vi "lab2(whithsubvi;works).vi"() -> ()   [LabVIEW 2016]
panel:
  out "2D Picture":picture
  in  "SwapGB":bool
  in  "SwapRB":bool
  in  "SwapRG":bool
  in  "Original":bool
  in  "ImagePath":path
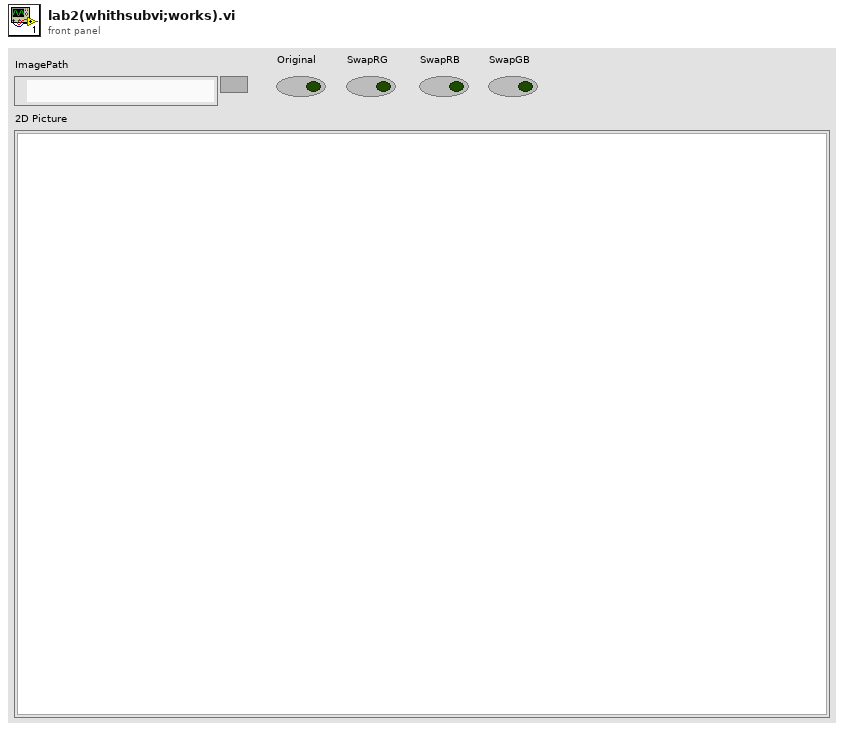
[diagram p1: front panel]
types:
  T1 = typedef "imagedata.ctl" = cluster{"image type":i32, "image depth":i32, "image":u8[], "mask":u8[], "colors":u32[], "Rectangle":cluster{"left":i16, "top":i16, "right":i16, "bottom":i16}}
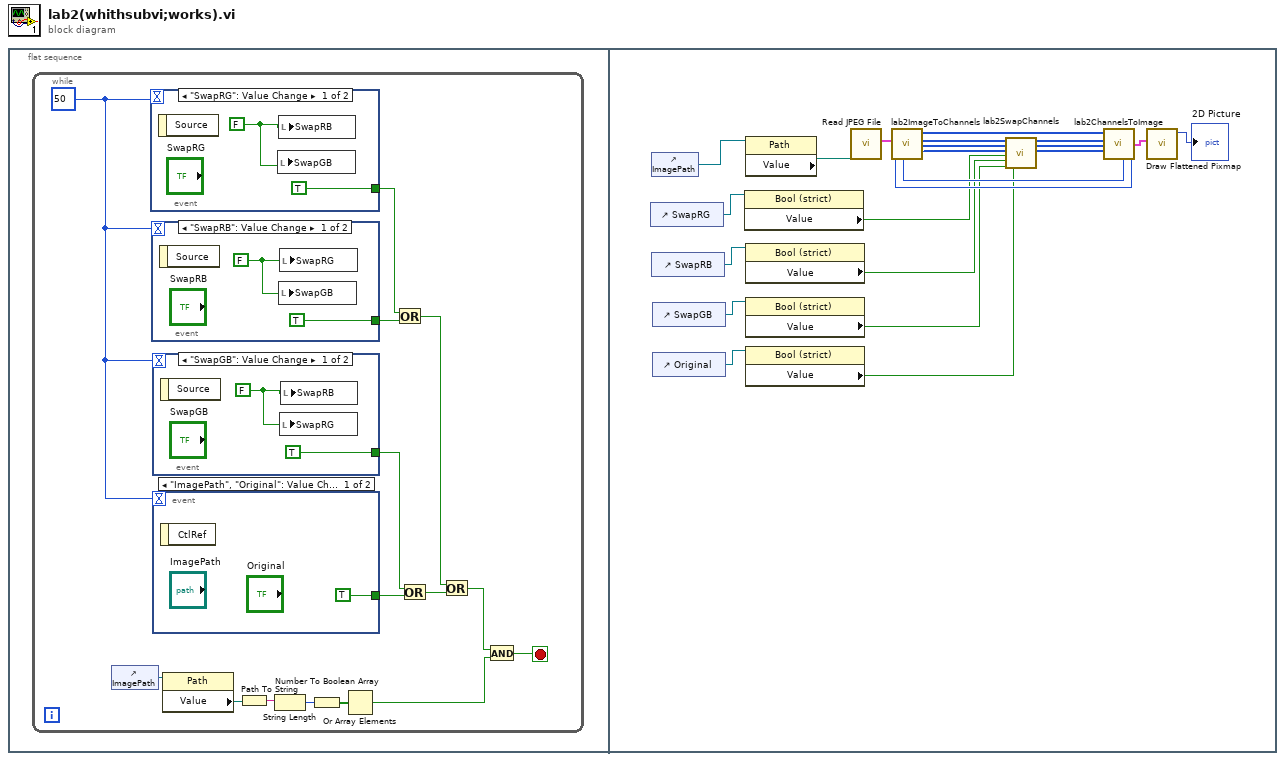
[diagram p0: block diagram]
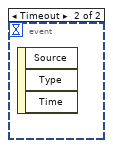
[diagram p2: hidden frame]
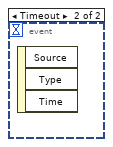
[diagram p3: hidden frame]
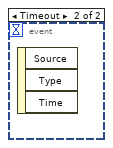
[diagram p4: hidden frame]
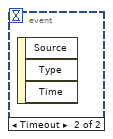
[diagram p5: hidden frame]
diagram:
  n1 = flat-sequence {
    frame #0 {
      n2 = while {
        stop <- w3 stop-if-true
        w11 = 50
        n3 = control-ref of="ImagePath"() -> (w15:refnum<vi>)
        n4 = event shown="[0] \"SwapRG\": Value Change" {
          selector: _ -> [_ _]
          dyn-events: _ -> [_ _]
          timeout: w11 -> [_ _]
          tunnel: [TRUE _] -> w5
          event "SwapRG": Value Change {
            w21 = FALSE
            n5 = event-data() -> ()  [unwired: 1 in, 1 out]
            n6 = local write "SwapGB"(w21) -> ()
            n7 = local write "SwapRB"(w21) -> ()
          }
          event Timeout {
            n8 = event-data() -> ()  [unwired: 1 in, 3 out]
          }
        }
        n9 = event shown="[0] \"SwapRB\": Value Change" {
          selector: _ -> [_ _]
          dyn-events: _ -> [_ _]
          timeout: w11 -> [_ _]
          tunnel: [TRUE _] -> w8
          event "SwapRB": Value Change {
            w19 = FALSE
            n10 = event-data() -> ()  [unwired: 1 in, 1 out]
            n11 = local write "SwapGB"(w19) -> ()
            n12 = local write "SwapRG"(w19) -> ()
          }
          event Timeout {
            n13 = event-data() -> ()  [unwired: 1 in, 3 out]
          }
        }
        n14 = event shown="[0] \"SwapGB\": Value Change" {
          selector: _ -> [_ _]
          dyn-events: _ -> [_ _]
          timeout: w11 -> [_ _]
          tunnel: [TRUE _] -> w4
          event "SwapGB": Value Change {
            w17 = FALSE
            n15 = event-data() -> ()  [unwired: 1 in, 1 out]
            n16 = local write "SwapRG"(w17) -> ()
            n17 = local write "SwapRB"(w17) -> ()
          }
          event Timeout {
            n18 = event-data() -> ()  [unwired: 1 in, 3 out]
          }
        }
        n19 = event shown="[0] \"ImagePath\", \"Original\": Value Change" {
          selector: _ -> [_ _]
          dyn-events: _ -> [_ _]
          timeout: w11 -> [_ _]
          tunnel: [TRUE _] -> w9
          event "ImagePath", "Original": Value Change {
            n20 = event-data() -> ()  [unwired: 1 in, 1 out]
          }
          event Timeout {
            n21 = event-data() -> ()  [unwired: 1 in, 3 out]
          }
        }
        n22 = property class="Path"(reference=w15) -> ("Value"=w14:path)  [unwired: 1 in, 2 out]
        n23 = Path To String(path=w14) -> (string=w13:string)
        n24 = String Length(string=w13) -> (length=w10:i32)
        n25 = Number To Boolean Array(number=w10) -> (Boolean array=w12:bool[])
        n26 = Or Array Elements(Boolean array=w12) -> (logical OR=w1:bool)
        n27 = Or(x=w5, y=w8) -> (x .or. y?=w6:bool)
        n28 = Or(x=w4, y=w9) -> (x .or. y?=w7:bool)
        n29 = Or(x=w6, y=w7) -> (x .or. y?=w2:bool)
        n30 = And(x=w2, y=w1) -> (x .and. y?=w3:bool)
      }
    }
    frame #1 {
      n31 = control-ref of="SwapRG"() -> (w35:refnum<vi>)
      n32 = control-ref of="ImagePath"() -> (w41:refnum<vi>)
      n33 = control-ref of="SwapRB"() -> (w34:refnum<vi>)
      n34 = control-ref of="SwapGB"() -> (w33:refnum<vi>)
      n35 = control-ref of="Original"() -> (w40:refnum<vi>)
      n36 = property class="Bool (strict)"(reference=w35) -> ("Value"=w29:bool)  [unwired: 1 in, 2 out]
      n37 = property class="Path"(reference=w41) -> ("Value"=w42:path)  [unwired: 1 in, 2 out]
      n38 = property class="Bool (strict)"(reference=w34) -> ("Value"=w28:bool)  [unwired: 1 in, 2 out]
      n39 = property class="Bool (strict)"(reference=w33) -> ("Value"=w27:bool)  [unwired: 1 in, 2 out]
      n40 = property class="Bool (strict)"(reference=w40) -> ("Value"=w26:bool)  [unwired: 1 in, 2 out]
      n41 = call <vilib>:"Read JPEG File.vi"("path to JPEG file"=w42) -> ("image data"=w44:T1)  [unwired: 8 in, 2 out]
      n42 = call "lab2ImageToChannels.vi"("image data"=w44) -> ("imgWidth"=w36:i32, "imgHeight"=w37:i32, "channel4"=w38:u8[], "redChannel"=w32:u8[], "greenChannel"=w31:u8[], "blueChannel"=w30:u8[])  [unwired: 2 in]
      n43 = call "lab2SwapChannels.vi"("redChannel in"=w32, "greenChannel in"=w31, "blueChannel in"=w30, "swapRg"=w29, "swapRb"=w28, "swapGb"=w27, "bypass"=w26) -> ("redChannel out"=w25:u8[], "greenChannel out"=w24:u8[], "blueChannel out"=w23:u8[])  [unwired: 10 in]
      n44 = call "lab2ChannelsToImage.vi"("imgWidth"=w36, "imgHeight"=w37, "blueChannel"=w23, "greenChannel"=w24, "redChannel"=w25, "channel4"=w38) -> ("image data"=w39:T1)  [unwired: 2 in]
      n45 = call <vilib>:"Draw Flattened Pixmap.vi"("image data"=w39) -> ("new picture"=→"2D Picture":picture)  [unwired: 8 in]
    }
  }
